vi "Test MQTT-3.1.2-2.vi"(8 "error in (no error)":errorcluster) -> (0 "error out":errorcluster)   [LabVIEW 2013]
uses:
  source/Control Packets/CONNACK/CONNACK.lvclass
  source/Control Packets/CONNACK/Connect Return Code -- enum.ctl
  source/Server/Connection/TCPConnection.lvclass
  source/Control Packets/CONNECT/CONNECT.lvclass
  source/Control Packets/ControlPacket/ControlPacket.lvclass
  <vilib>/addons/_JKI Toolkits/Caraya/classes/Test/Test.lvclass
  source/Control Packets/DISCONNECT/DISCONNECT.lvclass
  <vilib>/addons/_JKI Toolkits/Caraya/classes/Assert/Assert.lvclass
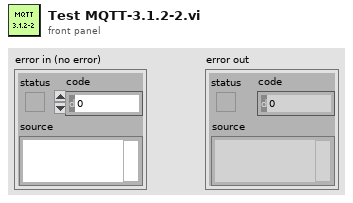
[diagram p1: front panel]
types:
  T1 = enum16{"Standard", "Buffered", "CRLF", "Immediate"}
  T2 = typedef "CONNACK.lvclass/Connect Return Code -- enum.ctl" = enum16{"Connection accepted", "Unacceptable protocol version", "Identifier Rejected", "Server Unavailable", "Bad Username or Password", "Not Authorized"}
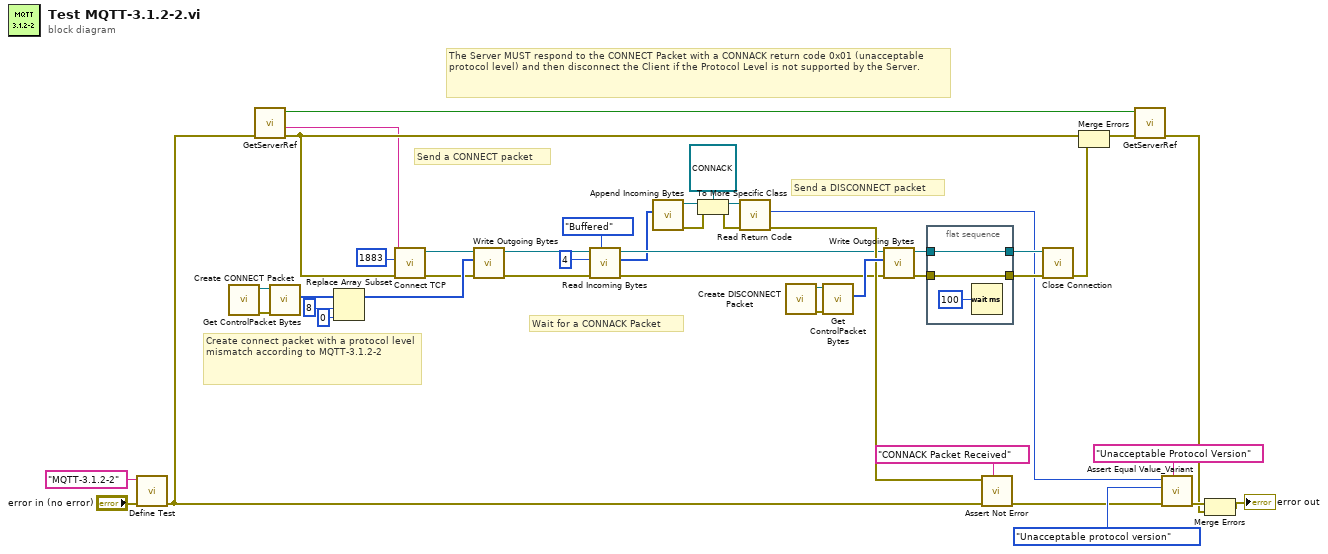
[diagram p0: block diagram]
diagram:
  # "The Server MUST respond to the CONNECT Packet with a CONNACK return code 0x01 (unacceptable protocol level) and then disconnect the Client if the Protocol Level is not supported by the Server."
  # "Send a DISCONNECT packet"
  # "Wait for a CONNACK Packet"
  # "Create connect packet with a protocol level mismatch according to MQTT-3.1.2-2"
  # "Send a CONNECT packet"
  n1 = call <vilib>:"Define Test.vi"("error in (no error)"="error in (no error)", "Label (VI Title)"="MQTT-3.1.2-2") -> ("error out"=w6:errorcluster)  [unwired: 9 in]
  n2 = call "Create CONNECT Packet.vi"() -> ("error out"=w44:errorcluster, "CONNECT"=w45:refnum<class "CONNECT.lvclass">)  [unwired: 10 in]
  n3 = call "GetServerRef.vi"("error in"=w6) -> ("error out"=w5:errorcluster, "Server address"=w2:string, "Created"=w7:bool)  [unwired: 7 in, 1 out]
  n4 = call "Get ControlPacket Bytes.vi"("error in (no error)"=w44, "ControlPacket"=w45) -> ("Bytes Stream"=w43:u8[])  [unwired: 7 in, 2 out]
  n5 = Replace Array Subset(array=w43, new element=u8 0 ("new element/subarray"), index=8) -> (w42:u8[])
  n6 = call "Connect TCP.vi"("error in (no error)"=w5, "remote port (80)"=u16 1883, "address (localhost)"=w2) -> ("error out"=w9:errorcluster, "TCPConnection out"=w10:refnum<class "TCPConnection.lvclass">)  [unwired: 7 in]
  n7 = call "Write Outgoing Bytes.vi"("error in (no error)"=w9, "Bytes"=w42, "TCPConnection in"=w10) -> ("error out"=w14:errorcluster, "TCPConnection out"=w15:refnum<class "TCPConnection.lvclass">)  [unwired: 7 in]
  n8 = call "Read Incoming Bytes.vi"("mode (standard)"=T1."Buffered", "error in (no error)"=w14, "bytes to read (100)"=4 ("bytes to read"), "TCPConnection in"=w15) -> ("error out"=w1:errorcluster, "Bytes"=w11:u8[], "TCPConnection out"=w12:refnum<class "TCPConnection.lvclass">)  [unwired: 4 in, 1 out]
  n9 = call "Append Incoming Bytes.vi"("Incoming Packets"=w11) -> ("error out"=w17:errorcluster, "ControlPacket"=w27:refnum<class "ControlPacket.lvclass">)  [unwired: 7 in, 2 out]
  n10 = To More Specific Class(target class=refnum<class "CONNACK.lvclass"> refnum ("CONNACK.lvclass"), reference=w27, error in=w17) -> (specific class reference=w25:refnum<class "CONNACK.lvclass">, error out=w21:errorcluster)
  n11 = call "Read Return Code.vi"("error in (no error)"=w21, "CONNACK in"=w25) -> ("error out"=w19:errorcluster, "Return Code"=w23:T2)  [unwired: 7 in, 1 out]
  n12 = call "Create DISCONNECT Packet.vi"() -> ("error out"=w35:errorcluster, "DISCONNECT"=w34:refnum<class "DISCONNECT.lvclass">)  [unwired: 10 in]
  n13 = call "Get ControlPacket Bytes.vi"("error in (no error)"=w35, "ControlPacket"=w34) -> ("Bytes Stream"=w33:u8[])  [unwired: 7 in, 2 out]
  n14 = call "Write Outgoing Bytes.vi"("error in (no error)"=w1, "Bytes"=w33, "TCPConnection in"=w12) -> ("error out"=w31:errorcluster, "TCPConnection out"=w32:refnum<class "TCPConnection.lvclass">)  [unwired: 7 in]
  n15 = flat-sequence {
    tunnel: w32 -> [w48]
    tunnel: [w48] -> w28
    tunnel: [w46] -> w24
    tunnel: w31 -> [w46]
    frame #0 {
      n16 = Wait (ms)(milliseconds to wait=u32 100) -> ()  [unwired: 1 out]
    }
  }
  n17 = call <vilib>:"Assert Not Error.vi"("Label"="CONNACK Packet Received", "error in (no error)"=w6, "Not Error?"=w19) -> ("error out"=w20:errorcluster)  [unwired: 8 in]
  n18 = call-dynamic "Close Connection.vi"("error in (no error)"=w24, "TCPConnection in"=w28) -> ("error out"=w37:errorcluster)  [unwired: 8 in, 1 out]
  n19 = Merge Errors(w5, w37) -> (w4:errorcluster)
  n20 = call "GetServerRef.vi"("error in"=w4, "Destroy (F)"=w7) -> ("error out"=w3:errorcluster)  [unwired: 6 in, 3 out]
  n21 = call <vilib>:"Assert Equal Value_Variant.vi"("Label"="Unacceptable Protocol Version", "error in (no error)"=w20, "Y"=Connect_Return_Code_--_enum."Unacceptable protocol version" ("Return Code"), "X"=w23) -> ("error out"=w40:errorcluster)  [unwired: 7 in]
  n22 = Merge Errors(w40, w3) -> (→"error out":errorcluster)
